vi "Send Command.vi"(6 "Command":T1, 8 "error in":errorcluster, 10 "Value":dbl, 11 "ThorlabsLabJack in":refnum<class "ThorlabsLabJack.lvclass">) -> (0 "error out":errorcluster, 3 "ThorlabsLabJack out":refnum<class "ThorlabsLabJack.lvclass">)   [LabVIEW 2018, in "ThorlabsLabJack.lvlib" / "ThorlabsLabJack.lvclass"]
doc: "This VI will send a specific command to the Motor."
uses:
  ThorlabsLabJack.lvclass
  PPLs/Axis/Parent/Axis.lvlibp/Custom Controls/Command.ctl
  PPLs/Axis/Parent/Axis.lvlibp
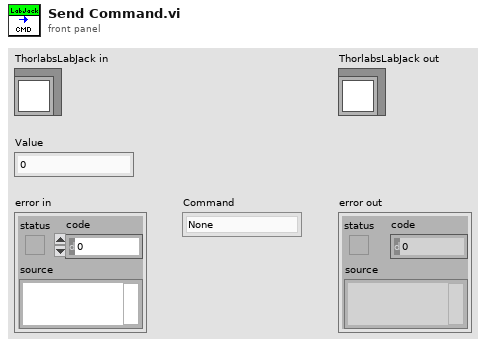
[diagram p1: front panel]
types:
  T1 = typedef "Axis.lvlibp/Command.ctl" = enum16{"None", "Home", "Renumber", "Move Absolute", "Move Relative", "Stop", "Set Run Speed", "Set Acceleration", "Set Run Current", "Set Home Offset", "Set Home Speed", "Query Current Position", "Load Defaults", "Query Status", "Lock Controls", "Unlock Controls", "Set Jog Step Size", "Set Jog Acceleration", "Set Jog Speed", "Query Homed Status", "Query Moving Status", "Reset", "Set Max Position", "Set Min Position"}
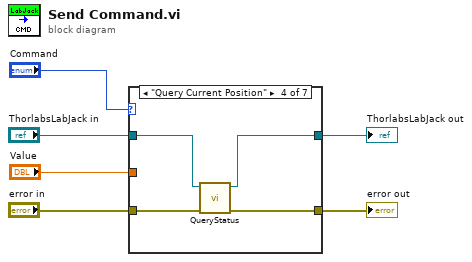
[diagram p0: block diagram]
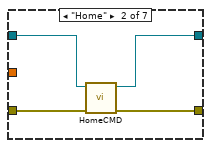
[diagram p3: hidden frame]
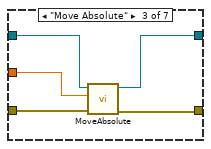
[diagram p4: hidden frame]
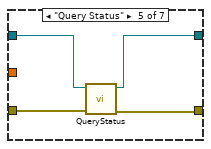
[diagram p5: hidden frame]
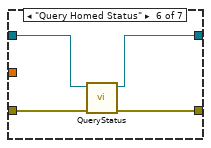
[diagram p6: hidden frame]
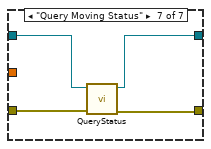
[diagram p7: hidden frame]
diagram:
  n1 = case shown="\"Query Current Position\"" "Command" {
    tunnel: "ThorlabsLabJack in" -> [w8 w10 w15 w18 w22 w29 w30]
    tunnel: "error in" -> [w7 w12 w17 w21 w25 w26 w33]
    tunnel: [w7 w11 w13 w20 w24 w27 w32] -> w3
    tunnel: [w8 w9 w14 w19 w23 w28 w31] -> w2
    tunnel: "Value" -> [_ _ w16 _ _ _ _]
    frame "None", Default {
    }
    frame "Home" {
      n2 = call "HomeCMD.vi"("error in (no error)"=w12, "ThorlabsLabJack in"=w10) -> ("error out"=w11:errorcluster, "ThorlabsLabJack out"=w9:refnum<class "ThorlabsLabJack.lvclass">)  [unwired: 8 in]
    }
    frame "Move Absolute" {
      n3 = call "MoveAbsolute.vi"("error in (no error)"=w17, "Move Abs Value"=w16, "ThorlabsLabJack in"=w15) -> ("error out"=w13:errorcluster, "ThorlabsLabJack out"=w14:refnum<class "ThorlabsLabJack.lvclass">)  [unwired: 7 in]
    }
    frame "Query Current Position" {
      n4 = call "QueryStatus.vi"("error in (no error)"=w21, "ThorlabsLabJack in"=w18) -> ("error out"=w20:errorcluster, "ThorlabsLabJack out"=w19:refnum<class "ThorlabsLabJack.lvclass">)  [unwired: 8 in]
    }
    frame "Query Status" {
      n5 = call "QueryStatus.vi"("error in (no error)"=w25, "ThorlabsLabJack in"=w22) -> ("error out"=w24:errorcluster, "ThorlabsLabJack out"=w23:refnum<class "ThorlabsLabJack.lvclass">)  [unwired: 8 in]
    }
    frame "Query Homed Status" {
      n6 = call "QueryStatus.vi"("error in (no error)"=w26, "ThorlabsLabJack in"=w29) -> ("error out"=w27:errorcluster, "ThorlabsLabJack out"=w28:refnum<class "ThorlabsLabJack.lvclass">)  [unwired: 8 in]
    }
    frame "Query Moving Status" {
      n7 = call "QueryStatus.vi"("error in (no error)"=w33, "ThorlabsLabJack in"=w30) -> ("error out"=w32:errorcluster, "ThorlabsLabJack out"=w31:refnum<class "ThorlabsLabJack.lvclass">)  [unwired: 8 in]
    }
  }
  "error out" <- w3
  "ThorlabsLabJack out" <- w2
